vi "traffic_signal(mini program).vi"() -> ()   [LabVIEW 2017]
panel:
  in  "布尔":bool
  out "green 4":bool
  out "yellow 4":bool
  out "red 4":bool
  out "green 3":bool
  out "yellow 3":bool
  out "red 3":bool
  out "green 2":bool
  out "yellow 2":bool
  out "red 2":bool
  out "green":bool
  out "yellow":bool
  out "red":bool
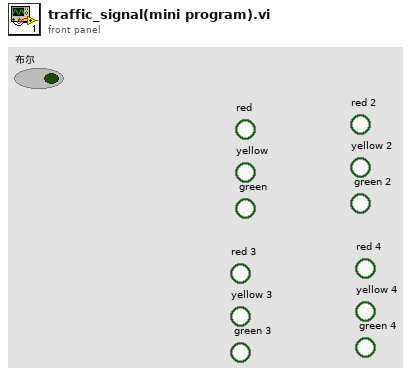
[diagram p1: front panel]
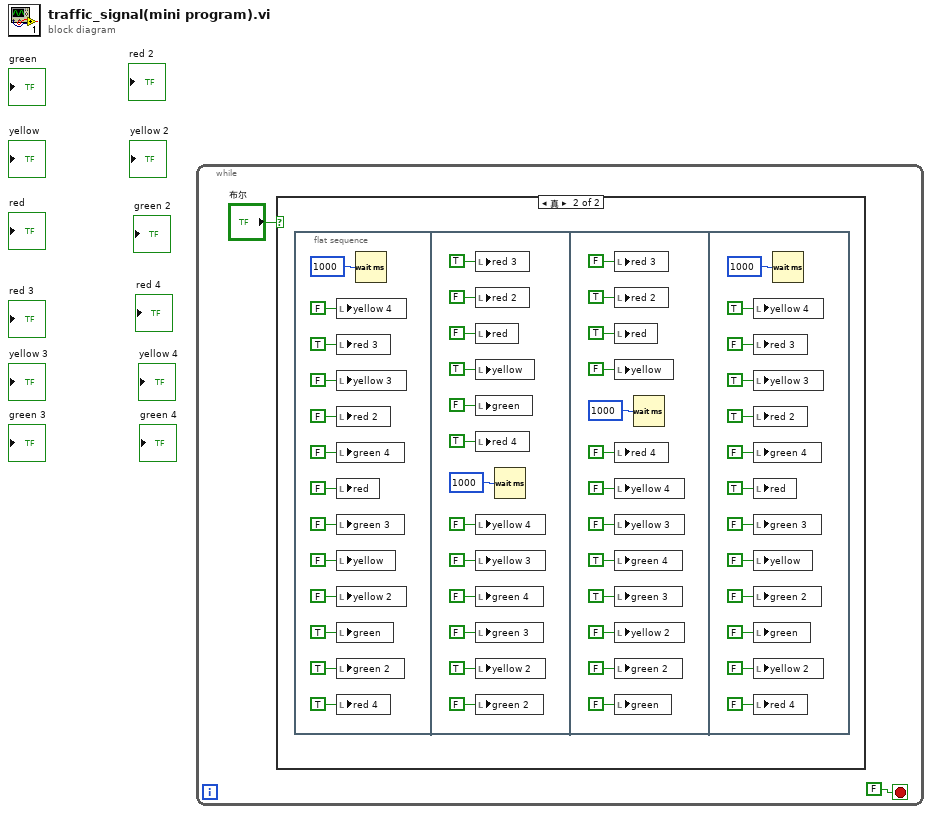
[diagram p0: block diagram]
diagram:
  n1 = while {
    stop <- FALSE stop-if-true
    n2 = case shown="真" "布尔" {
      frame False {
      }
      frame True {
        n3 = flat-sequence {
          frame #0 {
            n4 = local write "yellow 4"(FALSE ("yellow 4")) -> ()
            n5 = local write "red 3"(TRUE ("red 3")) -> ()
            n6 = local write "yellow 3"(FALSE ("yellow 3")) -> ()
            n7 = local write "red 2"(FALSE ("red 2")) -> ()
            n8 = local write "green 4"(FALSE ("green 4")) -> ()
            n9 = local write "red"(FALSE ("red")) -> ()
            n10 = local write "green 3"(FALSE ("green 3")) -> ()
            n11 = local write "yellow"(FALSE ("yellow")) -> ()
            n12 = local write "yellow 2"(FALSE ("yellow 2")) -> ()
            n13 = local write "green"(TRUE ("green")) -> ()
            n14 = local write "green 2"(TRUE ("green 2")) -> ()
            n15 = local write "red 4"(TRUE ("red 4")) -> ()
            n16 = Wait (ms)(milliseconds to wait=u32 1000 ("等待时间（毫秒）")) -> ()  [unwired: 1 out]
          }
          frame #1 {
            n17 = local write "red 3"(TRUE ("red 3")) -> ()
            n18 = local write "red 2"(FALSE ("red 2")) -> ()
            n19 = local write "red"(FALSE ("red")) -> ()
            n20 = local write "yellow"(TRUE ("yellow")) -> ()
            n21 = local write "green"(FALSE ("green")) -> ()
            n22 = local write "red 4"(TRUE ("red 4")) -> ()
            n23 = local write "yellow 4"(FALSE ("yellow 4")) -> ()
            n24 = local write "yellow 3"(FALSE ("yellow 3")) -> ()
            n25 = local write "green 4"(FALSE ("green 4")) -> ()
            n26 = local write "green 3"(FALSE ("green 3")) -> ()
            n27 = local write "yellow 2"(TRUE ("yellow 2")) -> ()
            n28 = local write "green 2"(FALSE ("green 2")) -> ()
            n29 = Wait (ms)(milliseconds to wait=u32 1000 ("等待时间（毫秒）")) -> ()  [unwired: 1 out]
          }
          frame #2 {
            n30 = local write "red 3"(FALSE ("red 3")) -> ()
            n31 = local write "red 2"(TRUE ("red 2")) -> ()
            n32 = local write "red"(TRUE ("red")) -> ()
            n33 = local write "yellow"(FALSE ("yellow")) -> ()
            n34 = local write "red 4"(FALSE ("red 4")) -> ()
            n35 = local write "yellow 4"(FALSE ("yellow 4")) -> ()
            n36 = local write "yellow 3"(FALSE ("yellow 3")) -> ()
            n37 = local write "green 4"(TRUE ("green 4")) -> ()
            n38 = local write "green 3"(TRUE ("green 3")) -> ()
            n39 = local write "yellow 2"(FALSE ("yellow 2")) -> ()
            n40 = local write "green 2"(FALSE ("green 2")) -> ()
            n41 = local write "green"(FALSE ("green")) -> ()
            n42 = Wait (ms)(milliseconds to wait=u32 1000 ("等待时间（毫秒）")) -> ()  [unwired: 1 out]
          }
          frame #3 {
            n43 = local write "yellow 4"(TRUE ("yellow 4")) -> ()
            n44 = local write "red 3"(FALSE ("red 3")) -> ()
            n45 = local write "yellow 3"(TRUE ("yellow 3")) -> ()
            n46 = local write "red 2"(TRUE ("red 2")) -> ()
            n47 = local write "green 4"(FALSE ("green 4")) -> ()
            n48 = local write "red"(TRUE ("red")) -> ()
            n49 = local write "green 3"(FALSE ("green 3")) -> ()
            n50 = local write "yellow"(FALSE ("yellow")) -> ()
            n51 = local write "green 2"(FALSE ("green 2")) -> ()
            n52 = local write "green"(FALSE ("green")) -> ()
            n53 = local write "yellow 2"(FALSE ("yellow 2")) -> ()
            n54 = local write "red 4"(FALSE ("red 4")) -> ()
            n55 = Wait (ms)(milliseconds to wait=u32 1000 ("等待时间（毫秒）")) -> ()  [unwired: 1 out]
          }
        }
      }
    }
  }
